vi "MtrPowerDigital.vi"(8 "PwrDwn":bool, 9 "PwrUp":bool, 11 "PwrON":bool) -> (3 "MtrPWR":dbl)   [LabVIEW 2015]
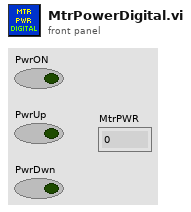
[diagram p1: front panel]
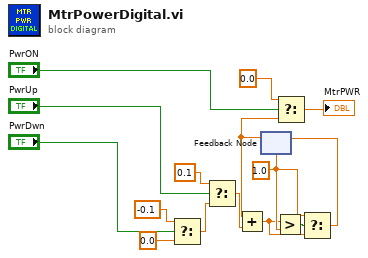
[diagram p0: block diagram]
diagram:
  w8 = 1.0
  n1 = Select(t=-0.1, s="PwrDwn", f=0.0) -> (s? t:f=w11:dbl)
  n2 = Select(t=0.1, s="PwrUp", f=w11) -> (s? t:f=w14:dbl)
  n3 = feedback #1(w8) -> (w13:dbl)
  n4 = Add(x=w13, y=w14) -> (x+y=w7:dbl)
  n5 = Greater?(x=w7, y=w8) -> (0:w9:bool)
  n6 = Select(t=0.0 ("Output"), s="PwrON", f=w13) -> (s? t:f=→"MtrPWR":dbl)
  n7 = Select(t=w8, s=w9, f=w7) -> (s? t:f=w6:dbl)
  n8 = feedback-in #1(w6) -> ()
